vi "Default Config--constant.vi"() -> (3 "Default Config":T1)   [LabVIEW 2023, in "VI Properties Editor.lvlib"]
doc: "Constant for the default config that will be written to the config for a user when the tool launches for the first time."
uses:
  VI Properties Editor.lvlib
  CTLs/Config.ctl
  <vilib>/Utility/sysdir.llb/System Directory Type.ctl
  CTLs/Filter Type.ctl
  CTLs/Column Name.ctl
  CTLs/Filter Info.ctl
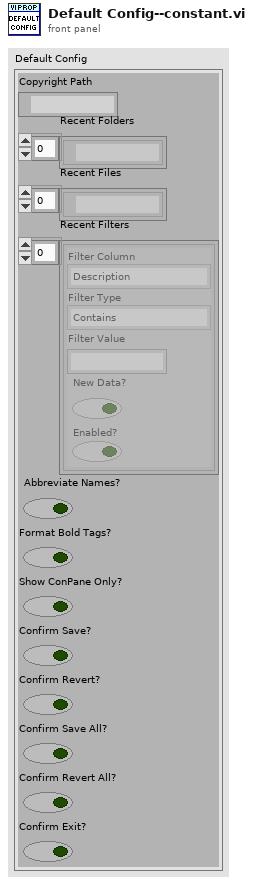
[diagram p1: front panel]
types:
  T1 = typedef "VI Properties Editor.lvlib/Config.ctl" = cluster{"Copyright Path":path, "Recent Folders":path[], "Recent Files":path[], "Recent Filters":T2[], "Abbreviate Names?":bool, "Format Bold Tags?":bool, "Show ConPane Only?":bool, "Confirm Save?":bool, "Confirm Revert?":bool, "Confirm Save All?":bool, "Confirm Revert All?":bool, "Confirm Exit?":bool}
  T2 = typedef "VI Properties Editor.lvlib/Filter Info.ctl" = cluster{"Filter Column":T3, "Filter Type":T4, "Filter Value":string, "New Data?":bool, "Enabled?":bool}
  T3 = typedef "VI Properties Editor.lvlib/Column Name.ctl" = enum16{"Name", "Path", "Type", "Window Title", "Description", "Help Path", "Help Tag", "Custom Title?", "Reentrant?", "Inlined?"}
  T4 = typedef "VI Properties Editor.lvlib/Filter Type.ctl" = enum16{"Contains", "Equals", "Starts with", "Ends with", "Does not contain", "Does not equal", "Is empty", "Is not empty"}
  T5 = typedef "System Directory Type.ctl" = i32
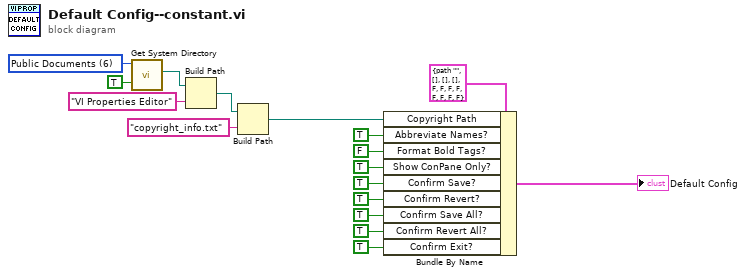
[diagram p0: block diagram]
diagram:
  w12 = T5 6 items=["User Home"=0, "User Desktop"=1, "User Documents"=2, "User Application Data"=3, "User Preferences"=4, "User Temporary"=5, "Public Documents"=6, "Public Application Data"=7, "Public Preferences"=8, "Public Cache"=13, "System Core Libraries"=9, "System Installed Libraries"=10, "Application Files"=11, "Boot Volume Root"=12] ("system directory type")
  n1 = call <vilib>:"Get System Directory.vi"("create directory if not found? (F)"=TRUE, "system directory type"=w12) -> ("system directory"=w14:path)  [unwired: 9 in]
  n2 = Build Path(base path=w14, name or relative path="VI Properties Editor") -> (appended path=w8:path)
  n3 = Build Path(base path=w8, name or relative path="copyright_info.txt") -> (appended path=w7:path)
  n4 = Bundle By Name(cluster=T1 {"Copyright Path"=path "", "Recent Folders"=[], "Recent Files"=[], "Recent Filters"=[], "Abbreviate Names?"=FALSE, "Format Bold Tags?"=FALSE, "Show ConPane Only?"=FALSE, "Confirm Save?"=FALSE, "Confirm Revert?"=FALSE, "Confirm Save All?"=FALSE, "Confirm Revert All?"=FALSE, "Confirm Exit?"=FALSE} ("Config"), "Copyright Path"=w7, "Abbreviate Names?"=TRUE, "Format Bold Tags?"=FALSE ("View Formatted Bold"), "Show ConPane Only?"=TRUE, "Confirm Save?"=TRUE ("Show Save Dialog?"), "Confirm Revert?"=TRUE ("Show Revert Dialog?"), "Confirm Save All?"=TRUE ("Show Save All Dialog?"), "Confirm Revert All?"=TRUE ("Show Revert All Dialog?"), "Confirm Exit?"=TRUE) -> (→"Default Config":T1)
